vi "calculate_scan_rate.vi"(8 "Scan rate number":dbl, 9 "Number of steps":dbl, 10 "Scan rate max (V/s)":dbl, 11 "Scan rate min (V/s)":dbl) -> (3 "Scan rate":dbl)   [LabVIEW 2016]
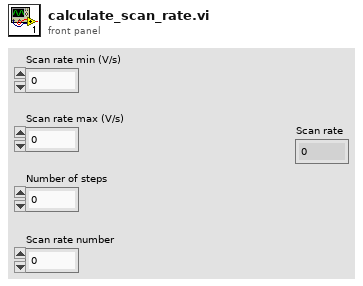
[diagram p1: front panel]
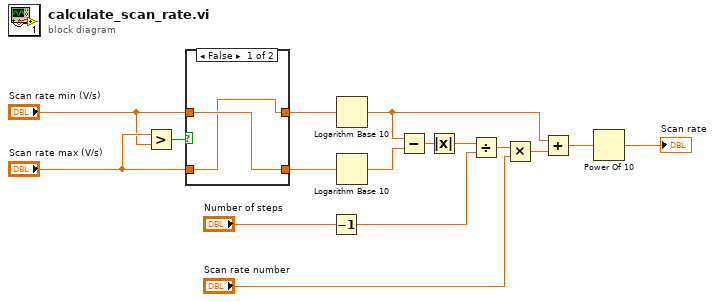
[diagram p0: block diagram]
diagram:
  n1 = Greater?(x="Scan rate max (V/s)", y="Scan rate min (V/s)") -> (0:w3:bool)
  n2 = case shown="False" w3 {
    tunnel: [w17 w20] -> w5
    tunnel: "Scan rate min (V/s)" -> [w18 w20]
    tunnel: [w18 w19] -> w4
    tunnel: "Scan rate max (V/s)" -> [w17 w19]
    frame False {
    }
    frame True {
    }
  }
  n3 = Decrement(x="Number of steps") -> (x-1=w12:dbl)
  n4 = Logarithm Base 10(1:w5) -> (0:w8:dbl)
  n5 = Logarithm Base 10(1:w4) -> (0:w16:dbl)
  n6 = Subtract(x=w8, y=w16) -> (x-y=w15:dbl)
  n7 = Absolute Value(x=w15) -> (abs(x)=w13:dbl)
  n8 = Divide(x=w13, y=w12) -> (x/y=w11:dbl)
  n9 = Multiply(x=w11, y="Scan rate number") -> (x*y=w9:dbl)
  n10 = Add(x=w8, y=w9) -> (x+y=w7:dbl)
  n11 = Power Of 10(x=w7) -> (10^x=→"Scan rate":dbl)
